vi "SMU Switch Handshaking - Advanced.vi"(4 "Source:Advanced:Source Delay":dbl=4e-05 format="%#_6p", 5 "Source:Transient Response":i32(ring)=1039 items=["Slow"=1041, "Normal"=1038, "Fast"=1039, "Custom"=1042], 7 "Measurement:Sense":i32(ring)=1008 items=["Local"=1008, "Remote"=1009], 8 "channels":string="0", 9 "Current":dbl=0.4 format="%#_6p", 10 "Voltage":dbl=0.6 format="%#_6p", 11 "resource name":refnum<k15>="SMU" caption="SMU resource name") -> (2 "R ch0":dbl=4.655063186197939e-06 format="%#_8p")   [LabVIEW 2018]
uses:
  <instrlib>/niSwitch/niSwitch.llb/niSwitch Topologies.ctl
  <instrlib>/niSwitch/niSwitch.llb/niSwitch Trigger Input.ctl
  <instrlib>/niSwitch/niSwitch.llb/niSwitch Scan Advanced Output.ctl
  <instrlib>/niDCPower/nidcpower.llb/niDCPower Export Signal - Signal.ctl
  <instrlib>/niDCPower/nidcpower.llb/niDCPower Wait For Event - Event.ctl
  <instrlib>/niDCPower/nidcpower.llb/niDCPower Configure Digital Edge Start Trigger.vi
  <instrlib>/niDCPower/nidcpower.llb/niDCPower Configure Digital Edge Sequence Advance Trigger.vi
  <vilib>/ptbypt/NI_PtbyPt.lvlib
panel:
  out "R ch5":dbl=5.495326889456616e-06 format="%#_8p"
  out "Waveform Chart ch5":dbl(graph)=5.495326889456616e-06
  out "standard deviation ch5":dbl=1.0083168978749402e-07 format="%.6p"
  out "R ch4":dbl=7.764040114943985e-06 format="%#_8p"
  out "Waveform Chart ch4":dbl(graph)=7.764040114943985e-06
  out "standard deviation ch4":dbl=1.0716800816728259e-07 format="%.6p"
  out "R ch3":dbl=0.6898081608102773 format="%#_8p"
  out "Waveform Chart ch3":dbl(graph)=0.6898081608102773
  out "standard deviation ch3":dbl=0.00017279619151355278 format="%.6p"
  out "R ch2":dbl=3.982851895772651e-06 format="%#_8p"
  out "Waveform Chart ch2":dbl(graph)=3.982851895772651e-06
  out "standard deviation ch2":dbl=1.2157242141278612e-07 format="%.6p"
  out "R ch1":dbl=4.419789069762714e-06 format="%#_8p"
  out "Waveform Chart ch1":dbl(graph)=4.419789069762714e-06
  out "standard deviation ch1":dbl=9.123309684182864e-08 format="%.6p"
  out "Elapsed Time (ms)":u32=6519
  in  "scan advanced output (External)":T1=enum."TTL1" caption="Scan Advanced Destination"
  in  "Trigger Source":T2=enum."TTL0"
  in  "topology name":T3="2530/1-Wire 4x32 Matrix" caption="Topology Name"
  in  "scan list":string="r0->c0&r1->c1&r2->c2&r3->c3;\nr0->c4&r1->c5&r2->c6&r3->c7;\nr0->c8&r1->c9&r2->c10&r3->c11;\nr0->c12&r1->c13&r2->c14&r3->c15;\nr0->c16&r1->c17&r2->c18&r3->c19;\nr0->c20&r1->c21&r2->c22&r3->c23;\n\n" caption="Scan List"
  in  "resource name 2":refnum<k15>="PXI1Slot5" caption="Switch Resource Name"
  in  "Measurement:Aperture Time":dbl=0.0833333 format="%#_6p"
  out "error out":errorcluster
  out "current measurements":dbl[](array[numeric])=[0.3999999889430746, -0.4000000709677936, -0.0009930024342528175, -0.0015522618824587338]
  out "voltage measurements":dbl[](array[numeric])=[1.5800847643981757e-05, 1.2614565888747521e-05, -4.6499699418282164e-05, -0.001065630272501495]
  in  "Measurement:Advanced:DC Noise Rejection":i32(ring)=1044 items=["Normal"=1044, "Second-Order"=1043]
  in  "Source:Advanced:Sequence Loop Count":i32=39
  out "standard deviation ch0":dbl=1.0919857002122854e-07 format="%.6p"
  out "Waveform Chart ch0":dbl(graph)=4.655063186197939e-06
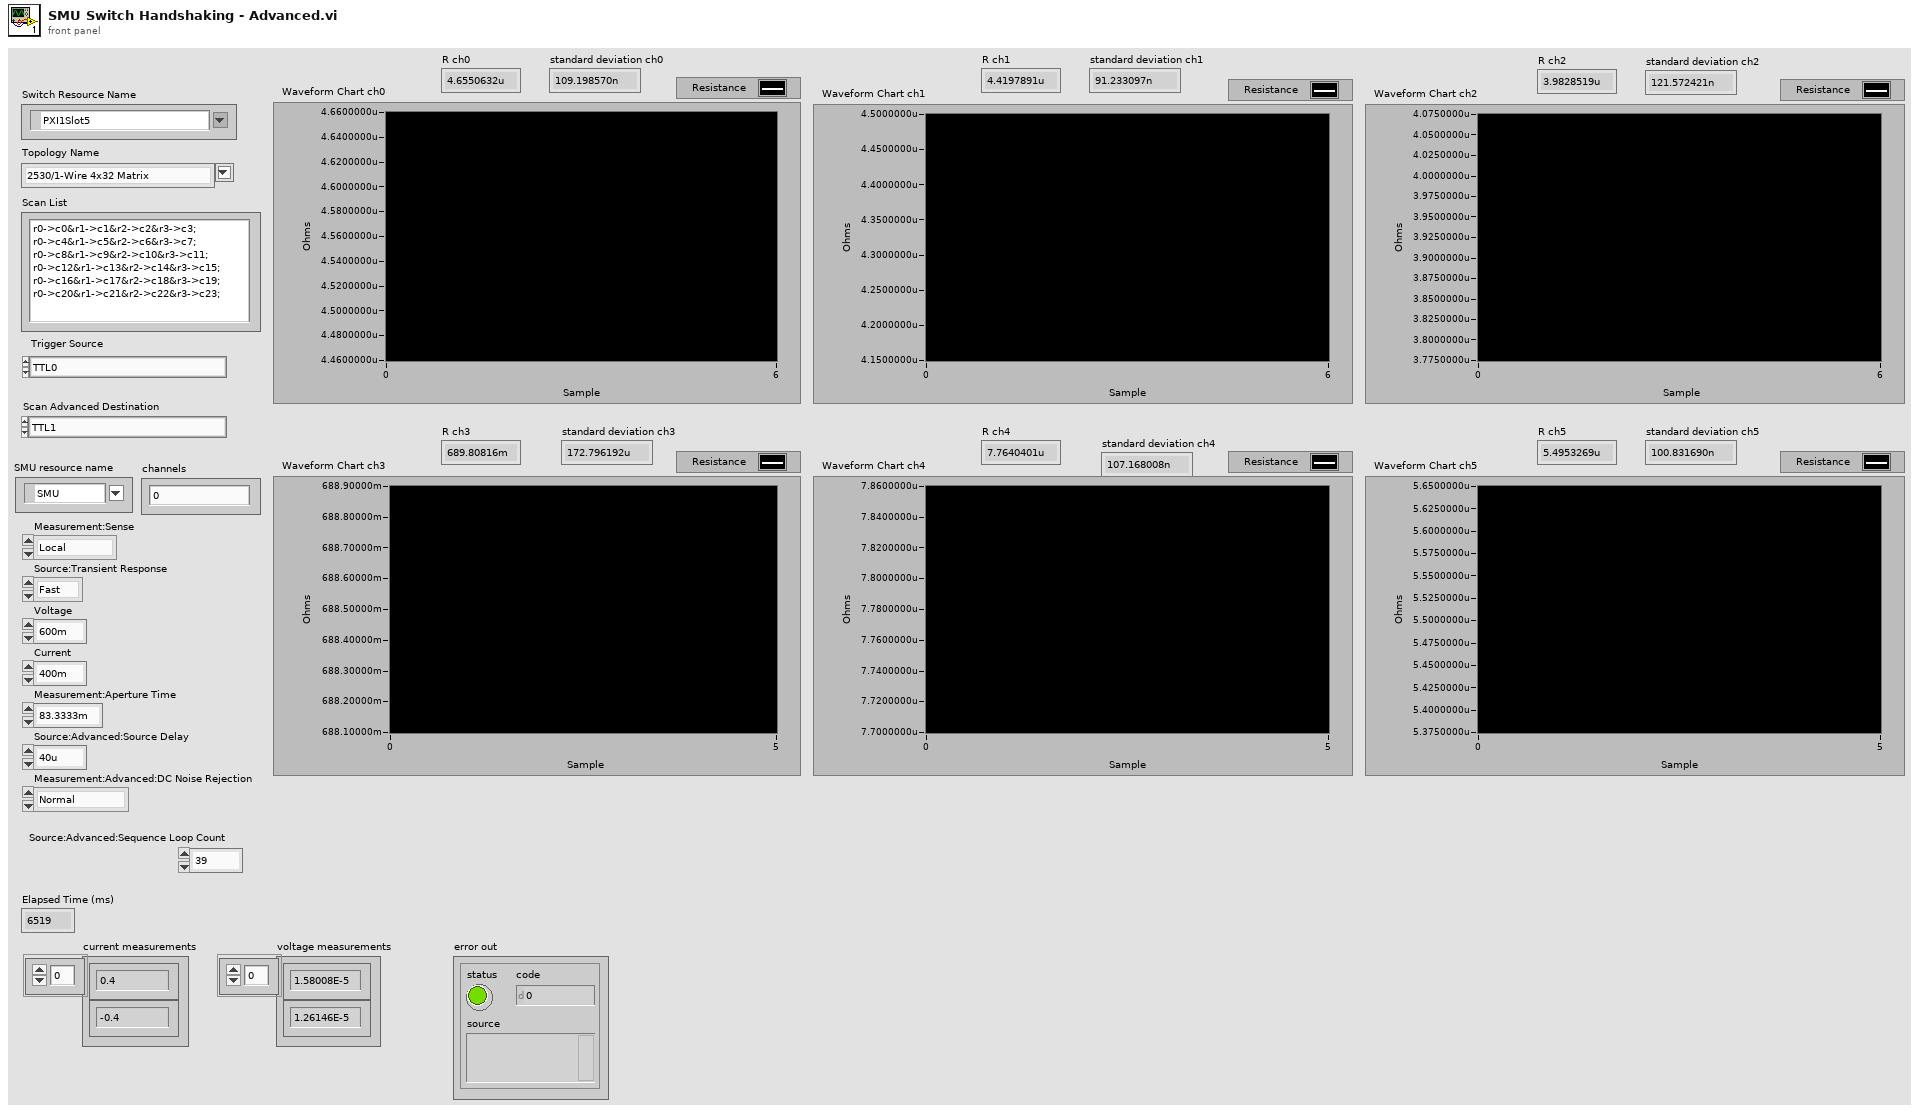
[diagram p1: front panel]
types:
  T1 = typedef "niSwitch Scan Advanced Output.ctl" = enum16{"None", "External", "TTL0", "TTL1", "TTL2", "TTL3", "TTL4", "TTL5", "TTL6", "TTL7", "ECL0", "ECL1", "PXI Star", "Rear Connector", "Front Connector", "Rear Connector Module 1", "Rear Connector Module 2", "Rear Connector Module 3", "Rear Connector Module 4", "Rear Connector Module 5", "Rear Connector Module 6", "Rear Connector Module 7", "Rear Connector Module 8", "Rear Connector Module 9", "Rear Connector Module 10", "Rear Connector Module 11", "Rear Connector Module 12", "Front Connector Module 1", "Front Connector Module 2", "Front Connector Module 3", "Front Connector Module 4", "Front Connector Module 5", "Front Connector Module 6", "Front Connector Module 7", "Front Connector Module 8", "Front Connector Module 9", "Front Connector Module 10", "Front Connector Module 11", "Front Connector Module 12"}
  T2 = typedef "niSwitch Trigger Input.ctl" = enum16{"Immediate", "External", "TTL0", "TTL1", "TTL2", "TTL3", "TTL4", "TTL5", "TTL6", "TTL7", "ECL0", "ECL1", "PXI Star", "Software Trigger Function", "Rear Connector", "Front Connector", "Rear Connector of Module 1", "Rear Connector of Module 2", "Rear Connector of Module 3", "Rear Connector of Module 4", "Rear Connector of Module 5", "Rear Connector of Module 6", "Rear Connector of Module 7", "Rear Connector of Module 8", "Rear Connector of Module 9", "Rear Connector of Module 10", "Rear Connector of Module 11", "Rear Connector of Module 12", "Front Connector of Module 1", "Front Connector of Module 2", "Front Connector of Module 3", "Front Connector of Module 4", "Front Connector of Module 5", "Front Connector of Module 6", "Front Connector of Module 7", "Front Connector of Module 8", "Front Connector of Module 9", "Front Connector of Module 10", "Front Connector of Module 11", "Front Connector of Module 12"}
  T3 = typedef "niSwitch Topologies.ctl" = string
  T4 = typedef "niDCPower Export Signal - Signal.ctl" = i32
  T5 = typedef "niDCPower Wait For Event - Event.ctl" = i32
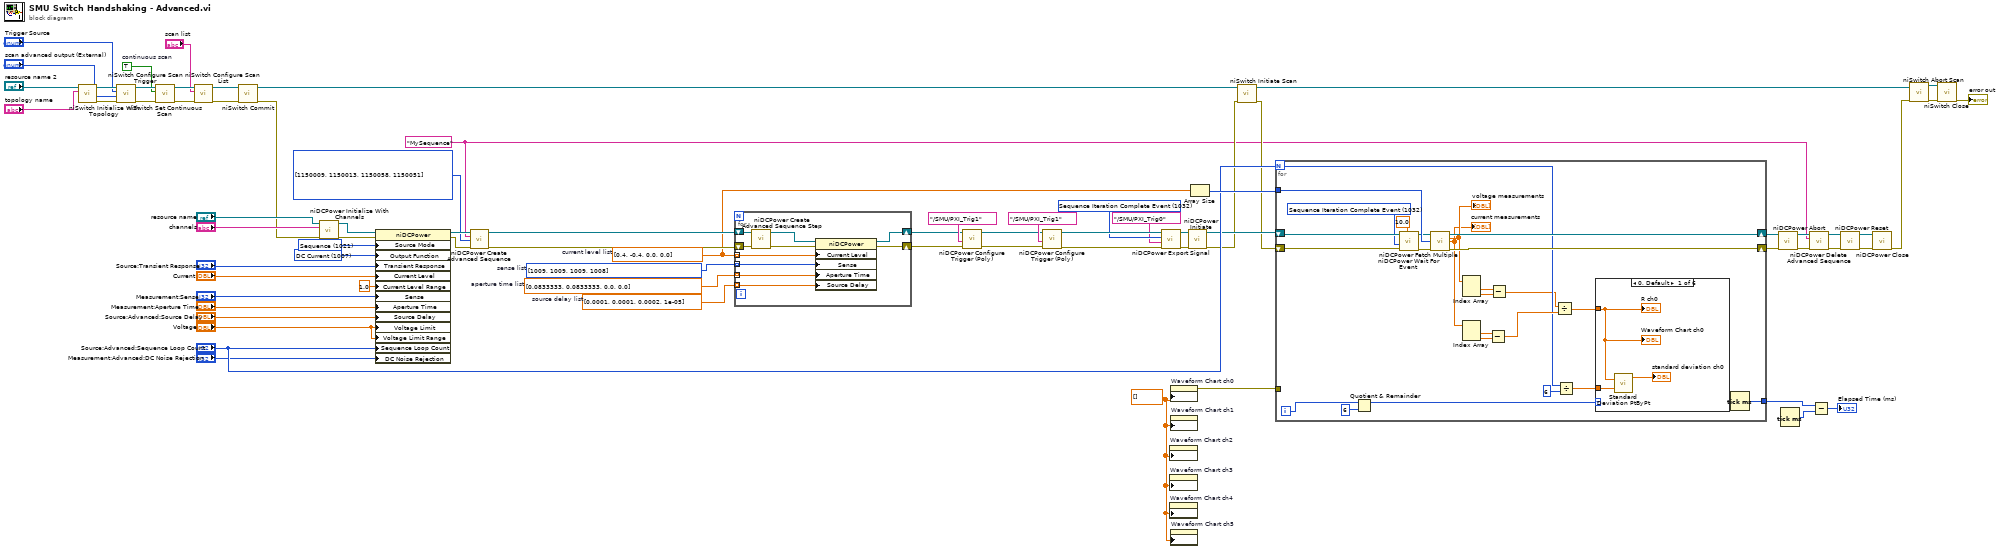
[diagram p0: block diagram]
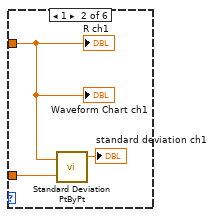
[diagram p2: hidden frame]
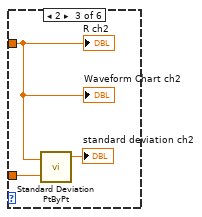
[diagram p3: hidden frame]
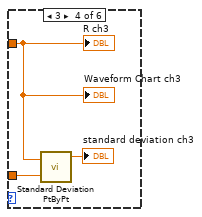
[diagram p4: hidden frame]
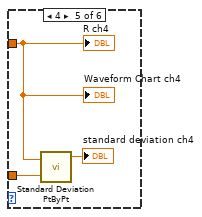
[diagram p5: hidden frame]
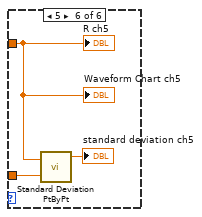
[diagram p6: hidden frame]
diagram:
  w1 = dbl[] [0.4, -0.4, 0.0, 0.0]  # current level list
  w6 = dbl[] [0.0833333, 0.0833333, 0.0, 0.0]  # aperture time list
  w5 = i32[] [1009, 1009, 1009, 1008] items=["Local"=1008, "Remote"=1009]  # sense list
  w9 = i32[] [1150009, 1150013, 1150058, 1150051] items=["Source -> Output Function"=1150008, "Source -> Output Enabled"=1250006, "Source -> Output Resistance"=1150061, "Source -> Transient Response"=1150062, "Source -> Custom Transient Response -> Voltage Gain Bandwidth"=1150067, "Source -> Custom Transient Response -> Voltage Compensation Frequency"=1150068, "Source -> Custom Transient Response -> Voltage Pole-Zero Ratio"=1150069, "Source -> Custom Transient Response -> Current Gain Bandwidth"=1150070, "Source -> Custom Transient Response -> Current Compensation Frequency"=1150071, "Source -> Custom Transient Response -> Current Pole-Zero Ratio"=1150072, "Source -> DC Voltage -> Voltage Level"=1250001, "Source -> DC Voltage -> Voltage Level Range"=1150005, "Source -> DC Voltage -> Current Limit"=1250005, "Source -> DC Voltage -> Current Limit High"=1150187, "Source -> DC Voltage -> Current Limit Low"=1150188, "Source -> DC Voltage -> Current Limit Range"=1150004, "Source -> DC Current -> Current Level"=1150009, "Source -> DC Current -> Current Level Range"=1150011, "Source -> DC Current -> Voltage Limit"=1150010, "Source -> DC Current -> Voltage Limit High"=1150185, "Source -> DC Current -> Voltage Limit Low"=1150186, "Source -> DC Current -> Voltage Limit Range"=1150012, "Source -> Pulse Voltage -> Pulse Voltage Level"=1150080, "Source -> Pulse Voltage -> Pulse Bias Voltage Level"=1150082, "Source -> Pulse Voltage -> Pulse Voltage Level Range"=1150084, "Source -> Pulse Voltage -> Pulse Current Limit"=1150081, "Source -> Pulse Voltage -> Pulse Current Limit High"=1150193, "Source -> Pulse Voltage -> Pulse Current Limit Low"=1150194, "Source -> Pulse Voltage -> Pulse Bias Current Limit"=1150083, "Source -> Pulse Voltage -> Pulse Bias Current Limit High"=1150195, "Source -> Pulse Voltage -> Pulse Bias Current Limit Low"=1150196, "Source -> Pulse Voltage -> Pulse Current Limit Range"=1150085, "Source -> Pulse Current -> Pulse Current Level"=1150086, "Source -> Pulse Current -> Pulse Bias Current Level"=1150088, "Source -> Pulse Current -> Pulse Current Level Range"=1150090, "Source -> Pulse Current -> Pulse Voltage Limit"=1150087, "Source -> Pulse Current -> Pulse Voltage Limit High"=1150189, "Source -> Pulse Current -> Pulse Voltage Limit Low"=1150190, "Source -> Pulse Current -> Pulse Bias Voltage Limit"=1150089, "Source -> Pulse Current -> Pulse Bias Voltage Limit High"=1150191, "Source -> Pulse Current -> Pulse Bias Voltage Limit Low"=1150192, "Source -> Pulse Current -> Pulse Voltage Limit Range"=1150091, "Source -> Advanced -> Source Delay"=1150051, "Source -> Advanced -> Pulse Bias Delay"=1150092, "Source -> Advanced -> Pulse On Time"=1150093, "Source -> Advanced -> Pulse Off Time"=1150094, "Source -> Advanced -> OVP Enabled"=1250002, "Source -> Advanced -> OVP Limit"=1250003, "Source -> Advanced -> Compliance Limit Symmetry"=1150184, "Source -> Advanced -> Sequence Step Delta Time"=1150198, "Measurement -> Sense"=1150013, "Measurement -> Aperture Time"=1150058, "Measurement -> Measure Record Length"=1150063, "Measurement -> Advanced -> DC Noise Rejection"=1150066] ("advanced sequence properties")
  w10 = "MySequence" ("sequence name")
  w26 = T4 1032 items=["Source Complete Event"=1030, "Measure Complete Event"=1031, "Sequence Iteration Complete Event"=1032, "Sequence Engine Done Event"=1033, "Pulse Complete Event"=1051, "Ready For Pulse Trigger Event"=1052, "Start Trigger"=1034, "Source Trigger"=1035, "Measure Trigger"=1036, "Sequence Advance Trigger"=1037, "Pulse Trigger"=1053] ("signal")
  w53 = TRUE  # continuous scan
  w4 = dbl[] [0.0001, 0.0001, 0.0002, 1e-05]  # source delay list
  w19 = dbl[] [] ("History Data")
  w74 = 1007 items=["DC Voltage"=1006, "DC Current"=1007, "Pulse Voltage"=1049, "Pulse Current"=1050] ("Source:Output Function")
  w75 = 1021 items=["Single Point"=1020, "Sequence"=1021] ("Source:Source Mode")
  n1 = call <instrlib>:"niSwitch Initialize With Topology.vi"("topology name"="topology name", "resource name"="resource name 2") -> ("error out"=w50:errorcluster, "instrument handle out"=w51:refnum<k15>)  [unwired: 3 in, 5 out]
  n2 = call <instrlib>:"niSwitch Configure Scan Trigger.vi"("error in (no error)"=w50, "scan advanced output (External)"="scan advanced output (External)", "trigger input (External)"="Trigger Source", "instrument handle"=w51) -> ("error out"=w54:errorcluster, "instrument handle out"=w56:refnum<k15>)  [unwired: 1 in, 5 out]
  n3 = call <instrlib>:"niSwitch Set Continuous Scan.vi"("error in (no error)"=w54, "continuous scan (False)"=w53, "instrument handle"=w56) -> ("error out"=w48:errorcluster, "instrument handle out"=w49:refnum<k15>)  [unwired: 7 out]
  n4 = call <instrlib>:"niSwitch Configure Scan List.vi"("error in (no error)"=w48, "scan list"="scan list", "instrument handle"=w49) -> ("error out"=w45:errorcluster, "instrument handle out"=w44:refnum<k15>)  [unwired: 1 in, 6 out]
  n5 = call <instrlib>:"niSwitch Commit.vi"("error in (no error)"=w45, "instrument handle"=w44) -> ("error out"=w38:errorcluster, "instrument handle out"=w43:refnum<k15>)  [unwired: 8 out]
  n6 = call <instrlib>:"niDCPower Initialize With Channels.vi"("error in (no error)"=w38, "channels"="channels", "resource name"="resource name") -> ("error out"=w68:errorcluster, "instrument handle out"=w69:refnum<k15>)  [unwired: 7 in]
  n7 = property class="niDCPower"(reference=w69, error in=w68, "Source Mode"=w75, "Output Function"=w74, "Transient Response"="Source:Transient Response", "Current Level"="Current", "Current Level Range"=1.0 ("Source:DC Current:Current Level Range"), "Sense"="Measurement:Sense", "Aperture Time"="Measurement:Aperture Time", "Source Delay"="Source:Advanced:Source Delay", "Voltage Limit"="Voltage", "Voltage Limit Range"="Voltage", "Sequence Loop Count"="Source:Advanced:Sequence Loop Count", "DC Noise Rejection"="Measurement:Advanced:DC Noise Rejection") -> (reference out=w18:refnum<k15>, error out=w17:errorcluster)
  n8 = call <instrlib>:"niDCPower Create Advanced Sequence.vi"("instrument handle"=w18, "sequence name"=w10, "advanced sequence properties"=w9, "error in (no error)"=w17) -> ("instrument handle out"=w8:refnum<k15>, "error out"=w7:errorcluster)  [unwired: 10 in]
  n9 = for {
    shift-right: [w82] -> w2
    shift-left: w7 -> [w85]
    shift-right: [w81] -> w3
    shift-left: w8 -> [w80]
    tunnel: w4 -> [w79] mode=indexing
    tunnel: w6 -> [w78] mode=indexing
    tunnel: w5 -> [w77] mode=indexing
    tunnel: w1 -> [w76] mode=indexing
    n10 = call <instrlib>:"niDCPower Create Advanced Sequence Step.vi"("error in (no error)"=w85, "instrument handle"=w80) -> ("error out"=w83:errorcluster, "instrument handle out"=w84:refnum<k15>)  [unwired: 8 in]
    n11 = property class="niDCPower"(reference=w84, error in=w83, "Current Level"=w76, "Sense"=w77, "Aperture Time"=w78, "Source Delay"=w79) -> (reference out=w81:refnum<k15>, error out=w82:errorcluster)
  }
  n12 = call-poly <instrlib>:"niDCPower Configure Trigger (Poly).vi"("error in (no error)"=w2, "input terminal"=tag "/SMU/PXI_Trig1", "instrument handle"=w3) -> ("error out"=w30:errorcluster, "instrument handle out"=w31:refnum<k15>)  [unwired: 7 in]
  n13 = call-poly <instrlib>:"niDCPower Configure Trigger (Poly).vi"("error in (no error)"=w30, "input terminal"=tag "/SMU/PXI_Trig1", "instrument handle"=w31) -> ("error out"=w25:errorcluster, "instrument handle out"=w27:refnum<k15>)  [unwired: 7 in]
  n14 = call <instrlib>:"niDCPower Export Signal.vi"("error in (no error)"=w25, "output terminal"=tag "/SMU/PXI_Trig0", "signal"=w26, "instrument handle"=w27) -> ("error out"=w28:errorcluster, "instrument handle out"=w29:refnum<k15>)  [unwired: 6 in]
  n15 = property on="Waveform Chart ch2" class="WFChart (strict)"("History Data"=w19) -> ()  [unwired: 2 in, 2 out]
  n16 = property on="Waveform Chart ch3" class="WFChart (strict)"("History Data"=w19) -> ()  [unwired: 2 in, 2 out]
  n17 = property on="Waveform Chart ch4" class="WFChart (strict)"("History Data"=w19) -> ()  [unwired: 2 in, 2 out]
  n18 = property on="Waveform Chart ch0" class="WFChart (strict)"("History Data"=w19) -> (error out=w63:errorcluster)  [unwired: 2 in, 1 out]
  n19 = property on="Waveform Chart ch1" class="WFChart (strict)"("History Data"=w19) -> ()  [unwired: 2 in, 2 out]
  n20 = property on="Waveform Chart ch5" class="WFChart (strict)"("History Data"=w19) -> ()  [unwired: 2 in, 2 out]
  n21 = call <instrlib>:"niDCPower Initiate.vi"("error in (no error)"=w28, "instrument handle"=w29) -> ("error out"=w37:errorcluster, "instrument handle out"=w57:refnum<k15>)  [unwired: 8 in]
  n22 = Array Size(array=w1) -> (size(s)=w70:i32)
  n23 = call <instrlib>:"niSwitch Initiate Scan.vi"("error in (no error)"=w37, "instrument handle"=w43) -> ("error out"=w36:errorcluster, "instrument handle out"=w46:refnum<k15>)  [unwired: 8 out]
  n24 = for {
    N: "Source:Advanced:Sequence Loop Count" -> [w90]
    tunnel: w70 -> [w110]
    shift-right: [w102] -> w61
    shift-left: w36 -> [w109]
    shift-right: [w103] -> w62
    shift-left: w57 -> [w108]
    tunnel: w63 -> [_]
    tunnel: [w94] -> w23
    i -> [w93]
    w107 = T5 1032 items=["Source Complete Event"=1030, "Measure Complete Event"=1031, "Sequence Iteration Complete Event"=1032, "Sequence Engine Done Event"=1033, "Pulse Complete Event"=1051, "Ready For Pulse Trigger Event"=1052] ("event")
    n25 = Quotient & Remainder(x=w93, y=6) -> (x-y*floor(x/y)=w91:i32)  [unwired: 1 out]
    n26 = call <instrlib>:"niDCPower Wait For Event.vi"("timeout (sec)"=10.0, "error in (no error)"=w109, "event"=w107, "instrument handle"=w108) -> ("error out"=w104:errorcluster, "instrument handle out"=w105:refnum<k15>)  [unwired: 6 in]
    n27 = call <instrlib>:"niDCPower Fetch Multiple.vi"("instrument handle"=w105, "count (1)"=w110, "error in (no error)"=w104) -> ("instrument handle out"=w103:refnum<k15>, "voltage measurements"=w101:dbl[], "current measurements"=w100:dbl[], "error out"=w102:errorcluster)  [unwired: 7 in, 2 out]
    "voltage measurements" <- w101
    "current measurements" <- w100
    n28 = Index Array(array=w101) -> (element #1=w99:dbl, element #2=w98:dbl)  [unwired: 2 in]
    n29 = Index Array(array=w100) -> (element #1=w97:dbl, element #2=w86:dbl)  [unwired: 2 in]
    n30 = Subtract(x=w97, y=w86) -> (x-y=w96:dbl)
    n31 = Subtract(x=w99, y=w98) -> (x-y=w87:dbl)
    n32 = Divide(x=w87, y=w96) -> (x/y=w95:dbl)
    n33 = Divide(x=w90, y=6) -> (x/y=w88:dbl)
    n34 = case shown="0, Default" w91 {
      tunnel: w95 -> [w112 w116 w118 w121 w124 w127]
      tunnel: w88 -> [w113 w115 w119 w122 w125 w128]
      frame 0, Default {
        n35 = call <vilib>:"Standard Deviation PtByPt.vi"("x"=w112, "sample length"=w113) -> ("standard deviation"=→"standard deviation ch0":dbl)  [unwired: 1 in, 2 out]
        "R ch0" <- w112
        "Waveform Chart ch0" <- w112
      }
      frame 1 {
        n36 = call <vilib>:"Standard Deviation PtByPt.vi"("x"=w116, "sample length"=w115) -> ("standard deviation"=→"standard deviation ch1":dbl)  [unwired: 1 in, 2 out]
        "R ch1" <- w116
        "Waveform Chart ch1" <- w116
      }
      frame 2 {
        n37 = call <vilib>:"Standard Deviation PtByPt.vi"("x"=w118, "sample length"=w119) -> ("standard deviation"=→"standard deviation ch2":dbl)  [unwired: 1 in, 2 out]
        "R ch2" <- w118
        "Waveform Chart ch2" <- w118
      }
      frame 3 {
        n38 = call <vilib>:"Standard Deviation PtByPt.vi"("x"=w121, "sample length"=w122) -> ("standard deviation"=→"standard deviation ch3":dbl)  [unwired: 1 in, 2 out]
        "R ch3" <- w121
        "Waveform Chart ch3" <- w121
      }
      frame 4 {
        n39 = call <vilib>:"Standard Deviation PtByPt.vi"("x"=w124, "sample length"=w125) -> ("standard deviation"=→"standard deviation ch4":dbl)  [unwired: 1 in, 2 out]
        "R ch4" <- w124
        "Waveform Chart ch4" <- w124
      }
      frame 5 {
        n40 = call <vilib>:"Standard Deviation PtByPt.vi"("x"=w127, "sample length"=w128) -> ("standard deviation"=→"standard deviation ch5":dbl)  [unwired: 1 in, 2 out]
        "R ch5" <- w127
        "Waveform Chart ch5" <- w127
      }
    }
    n41 = Tick Count (ms)() -> (millisecond timer value=w94:u32)
  }
  n42 = call <instrlib>:"niDCPower Abort.vi"("error in (no error)"=w61, "instrument handle"=w62) -> ("error out"=w15:errorcluster, "instrument handle out"=w16:refnum<k15>)  [unwired: 8 in]
  n43 = Tick Count (ms)() -> (millisecond timer value=w22:u32)
  n44 = call <instrlib>:"niDCPower Delete Advanced Sequence.vi"("error in (no error)"=w15, "sequence name"=w10, "instrument handle"=w16) -> ("error out"=w14:errorcluster, "instrument handle out"=w13:refnum<k15>)  [unwired: 7 in]
  n45 = Subtract(x=w23, y=w22) -> (x-y=→"Elapsed Time (ms)":u32)
  n46 = call <instrlib>:"niDCPower Reset.vi"("error in (no error)"=w14, "instrument handle"=w13) -> ("error out"=w11:errorcluster, "instrument handle out"=w12:refnum<k15>)  [unwired: 2 in, 6 out]
  n47 = call <instrlib>:"niDCPower Close.vi"("error in (no error)"=w11, "instrument handle"=w12) -> ("error out"=w35:errorcluster)  [unwired: 9 in]
  n48 = call <instrlib>:"niSwitch Abort Scan.vi"("error in (no error)"=w35, "instrument handle"=w46) -> ("error out"=w52:errorcluster, "instrument handle out"=w55:refnum<k15>)  [unwired: 8 out]
  n49 = call <instrlib>:"niSwitch Close.vi"("error in (no error)"=w52, "instrument handle"=w55) -> ("error out"=→"error out":errorcluster)  [unwired: 9 out]
